vi "Append.vi"   [LabVIEW 2016, in "xy_utilities.lvlib"]
doc: "Append <B>XY-Data B</B> to the end of <B>XY-Data A</B> (similar to Append Waveforms.vi).\n\nWire data to the data input to determine the polymorphic instance to use or manually select the instance."
uses:
  xy_utilities.lvlib
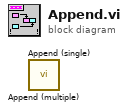
[diagram p0: block diagram]
diagram:
  n1 = call "Append (multiple).vi"() -> ()  [unwired: 10 in, 2 out]
  n2 = call "Append (single).vi"() -> ()  [unwired: 10 in, 2 out]
